vi "Start New Report.vi"(8 "error in (no error)":errorcluster, 9 "Report Path":path, 11 "ResultProcessor in":refnum<class "ResultProcessor.lvclass">) -> (0 "error out":errorcluster, 3 "ResultProcessor out":refnum<class "ResultProcessor.lvclass">)   [LabVIEW 2015, in "ResultProcessor.lvclass"]
doc: "This VI will start a new report. If a previous report was in progress and you have not called Publish Report, you will lose that previous report."
uses:
  ResultProcessor.lvclass
  CommandQueueDataType.ctl
  Report Information/Report Information.lvclass
  Result/Result.lvclass
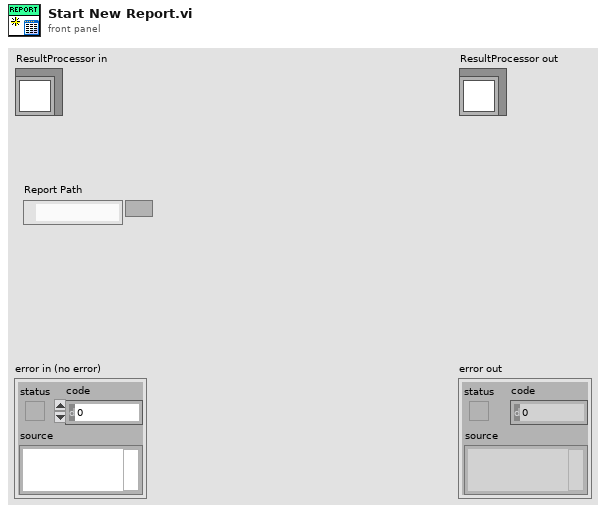
[diagram p1: front panel]
types:
  T1 = typedef "ResultProcessor.lvclass/CommandQueueDataType.ctl" = cluster{"Command":enum16{"New Report", "Add Result", "Publish Report", "Shutdown", "Add DUT Information", "Add Station Information", "Add Report Information", "Add Test Information"}, "Report Information.lvclass":refnum<class "Report Information.lvclass">, "Result.lvclass":refnum<class "Result.lvclass">}
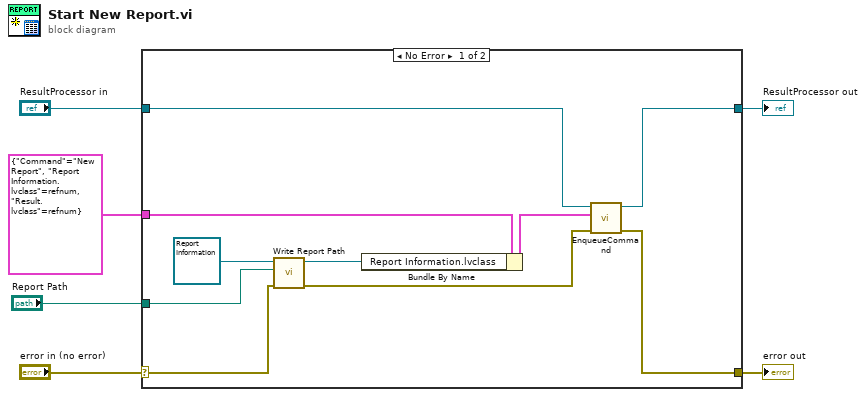
[diagram p0: block diagram]
diagram:
  n1 = case shown="No Error" "error in (no error)" {
    selector: "error in (no error)" -> [w10 w18]
    tunnel: [w14 w18] -> w5
    tunnel: [w15 w17] -> w3
    tunnel: "ResultProcessor in" -> [w16 w17]
    tunnel: T1 {"Command"=enum."New Report", "Report Information.lvclass"=refnum, "Result.lvclass"=refnum} ("element") -> [w13 _]
    tunnel: "Report Path" -> [w11 _]
    frame No Error {
      n2 = call-dynamic "Write Report Path.vi"("error in (no error)"=w10, "Report Path"=w11, "Report Information in"=refnum<class "Report Information.lvclass"> refnum ("Report Information.lvclass")) -> ("error out"=w9:errorcluster, "Report Information out"=w7:refnum<class "Report Information.lvclass">)  [unwired: 7 in]
      n3 = Bundle By Name(cluster=w13, "Report Information.lvclass"=w7) -> (w8:T1)
      n4 = call "EnqueueCommand.vi"("error in (no error)"=w9, "element"=w8, "ResultProcessor in"=w16) -> ("error out"=w14:errorcluster, "ResultProcessor out"=w15:refnum<class "ResultProcessor.lvclass">)  [unwired: 7 in]
    }
    frame Error {
    }
  }
  "error out" <- w5
  "ResultProcessor out" <- w3
